vi "LJUD_eTCConfigSB.vi"(0 "Handle In":i32, 1 "aEnableCounters":bool[](array[boolean]), 5 "aEnableTimers":bool[](array[boolean]), 7 "aTimerModes":string[](array[string]), 9 "aTimerValues":dbl[](array[numeric]) format="%.2f", 11 "error in":errorcluster, 12 "TCPinOffset":i32, 13 "TimerClockBase":string="LJ_tcSYS", 14 "TimerClockDivisor":i32) -> (4 "Handle Out":i32, 15 "error out":errorcluster)   [LabVIEW 2021]
doc: "This is an e-function that can configure\nand initialize all the timers and counters\nin a single call. A somewhat complex\nfunction, but can help reinforce the\ninteraction between the different timers\nand counters on the device.\n\nSee Sections 4.2 and 4.3 of the device's\ndatasheet for more information."
uses:
  labjackud.dll
panel:
  # "This version of eTCConfig uses\nstrings and booleans for some\nparameters.  This makes for more\nreadable programs."
  # "TimerClockBase Strings:\n\nU3 V1.20:\nLJ_tc2MHZ\nLJ_tc6MHZ\nLJ_tc24MHZ\nLJ_tc500KHZ_DIV\nLJ_tc2MHZ_DIV\nLJ_tc6MHZ_DIV\nLJ_tc24MHZ_DIV\n\nU6 and U3 V1.21+:\nLJ_tc4MHZ\nLJ_tc12MHZ\nLJ_tc48MHZ\nLJ_tc1MHZ_DIV\nLJ_tc4MHZ_DIV\nLJ_tc12MHZ_DIV\nLJ_tc48MHZ_DIV\nLJ_tcSYS    //48MHz\n\nUE9:\nLJ_tc750KHZ\nLJ_tcSYS     //48MHz"
  # "This is an e-function that can configure\nand initialize all the timers and counters\nin a single call.  A somewhat complex\nfunction, but can help reinforce the\ninteraction between the different timers\nand counters on the device.\n\nSee Sections 4.2 and 4.3 of the device's\ndatasheet for more information."
  # "Timer Mode Strings:\nLJ_tmPWM16\nLJ_tmPWM8\nLJ_tmRISINGEDGES32\nLJ_tmFALLINGEDGES32\nLJ_tmDUTYCYCLE\nLJ_tmFIRMCOUNTER\nLJ_tmFIRMCOUNTERDEBOUNCE\nLJ_tmFREQOUT\nLJ_tmQUAD\nLJ_tmTIMERSTOP\nLJ_tmSYSTIMERLOW\nLJ_tmSYSTIMERHIGH\nLJ_tmRISINGEDGES16\nLJ_tmFALLINGEDGES16\nLJ_tmLINETOLINE"
  # "Must be enabled\nsequentially."
  # "(0-255 where 0=256)"
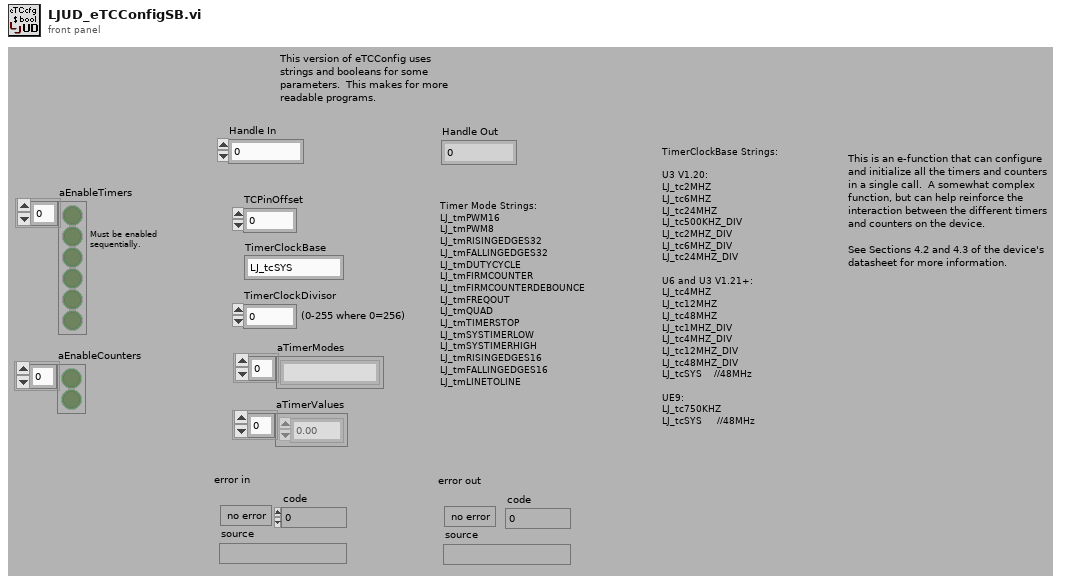
[diagram p1: front panel]
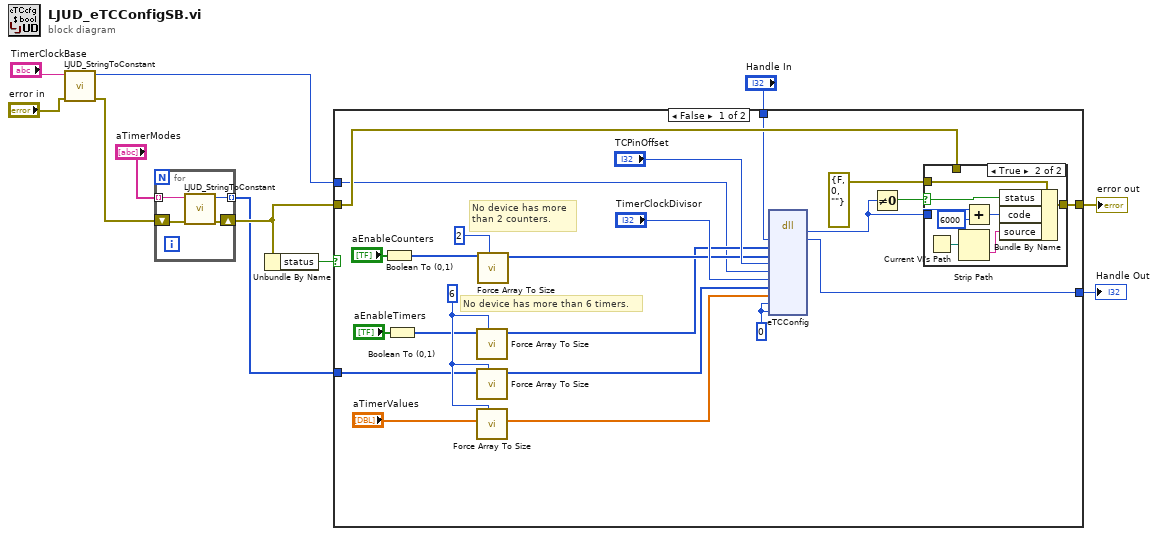
[diagram p0: block diagram]
diagram:
  n1 = call "LJUD_StringToConstant.vi"("error in"="error in", "String"="TimerClockBase") -> ("error out"=w7:errorcluster, "Constant Number"=w5:i32)  [unwired: 8 in]
  n2 = for {
    tunnel: "aTimerModes" -> [w15] mode=indexing
    shift-right: [w13] -> w6
    shift-left: w7 -> [w14]
    tunnel: [w12] -> w4 mode=indexing
    n3 = call "LJUD_StringToConstant.vi"("error in"=w14, "String"=w15) -> ("error out"=w13:errorcluster, "Constant Number"=w12:i32)  [unwired: 8 in]
  }
  n4 = Unbundle By Name(w6) -> ("status"=w10:bool)
  n5 = case shown="False" w10 {
    tunnel: [w35 w49] -> w11
    tunnel: w6 -> [w34 w49]
    tunnel: w5 -> [w23 _]
    tunnel: w4 -> [w22 _]
    tunnel: "Handle In" -> [w17 w48]
    tunnel: [w16 w48] -> w1
    frame False {
      w24 = 6 ("# Elements")
      w31 = 0 ("GoError")
      # "No device has more than 6 timers."
      # "No device has more\nthan 2 counters."
      n6 = Boolean To (0,1)(Boolean="aEnableCounters") -> (0, 1=w19:i16[])
      n7 = Boolean To (0,1)(Boolean="aEnableTimers") -> (0, 1=w18:i16[])
      n8 = call "Force Array To Size.vi"("# Elements"=w24, "I32 Array In"=w18) -> ("I32 Array Out"=w25:i32[])  [unwired: 6 in, 3 out]
      n9 = call "Force Array To Size.vi"("# Elements"=w24, "I32 Array In"=w22) -> ("I32 Array Out"=w26:i32[])  [unwired: 6 in, 3 out]
      n10 = call "Force Array To Size.vi"("# Elements"=w24, "DBL Array In"="aTimerValues") -> ("DBL Array Out"=w27:dbl[])  [unwired: 6 in, 3 out]
      n11 = call "Force Array To Size.vi"("# Elements"=2, "I32 Array In"=w19) -> ("I32 Array Out"=w30:i32[])  [unwired: 6 in, 3 out]
      n12 = dll-call lib="labjackud.dll" fn="eTCConfig"("Handle"=w17, "aEnableTimers"=w25, "aEnableCounters"=w30, "TCPinOffset"="TCPinOffset", "TimerClockBaseIndex"=w23, "TimerClockDivisor"="TimerClockDivisor", "aTimerModes"=w26, "aTimerValues"=w27, "Reserved1"=w31, "Reserved2"=w31) -> (w36:i32, "Handle"=w16:i32)  [unwired: 12 in, 2 out]
      n13 = Not Equal To 0?(x=w36) -> (x != 0?=w37:bool)
      n14 = case shown="True" w37 {
        selector: w37 -> [_ w46]
        tunnel: [w39 w47] -> w35
        tunnel: errorcluster {"status"=FALSE, "code"=0, "source"=""} ("error IO") -> [_ w45]
        tunnel: w36 -> [_ w41]
        tunnel: w34 -> [w39 _]
        frame False {
        }
        frame True {
          n15 = Current VI's Path() -> (path=w43:path)
          n16 = Strip Path(path=w43) -> (name=w44:string)  [unwired: 1 out]
          n17 = Add(x=w41, y=6000) -> (x+y=w42:i32)
          n18 = Bundle By Name(cluster=w45, "status"=w46, "code"=w42, "source"=w44) -> (w47:errorcluster)
        }
      }
    }
    frame True {
    }
  }
  "error out" <- w11
  "Handle Out" <- w1
